vi "CreatePrivateEvents.vi"(8 "error in (no error)":errorcluster, 11 "SignalSenderLoop":refnum<class "SignalSenderLoop.lvclass">) -> (0 "error out":errorcluster, 3 "SignalSenderLoop out":refnum<class "SignalSenderLoop.lvclass">)   [LabVIEW 2020, in "SignalSenderLoop.lvclass"]
doc: "JKI State Machine Objects (SMO) 1.1.0.20\nJKI - JKI\nCopyright (c) 2016, JKI"
uses:
  SignalSenderLoop.lvclass
  SignalSenderLoop.lvclass/SignalSenderLoop.ctl
  Typedefs/AsyncMethodInputs--Cluster.ctl
  Typedefs/PrivateEvents--SignalSenderLoop.SignalCMDArry.ctl
  <vilib>/JKI/JKI SMO/SMO/SMO.lvclass
panel:
  # "For instructions on how to use the JKI State Machine Objects, examples and video tutorials, visit:\nhttp://jki.net/state-machine-objects/\n\nJKI State Machine Objects™\nhttp://jki.net/state-machine-objects/\nCopyright (C) 2005-2015, JKI <info@jki.net>\nALL RIGHTS RESERVED"
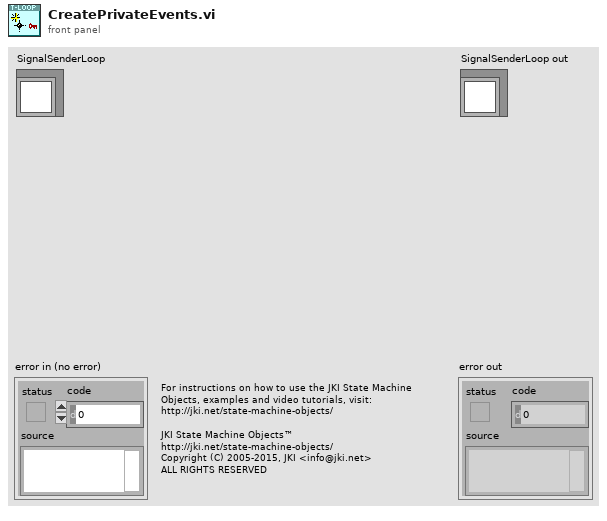
[diagram p1: front panel]
types:
  T1 = typedef "SignalSenderLoop.lvclass/PrivateData--Ref.ctl" = refnum<data-value>
  T2 = typedef "SignalSenderLoop.lvclass/PrivateEvents--SignalSenderLoop.SignalCMDArry.ctl" = dbl[]
  T3 = typedef "SignalSenderLoop.lvclass/AsyncMethodInputs--Cluster.ctl" = cluster{"Data":dbl}
  T4 = typedef "SignalSenderLoop.lvclass/PrivateData--Cluster.ctl" = cluster{"Public Events":T5, "Setpoint":T6, "Private Events":T7, "SignalFrameSet":T8}
  T5 = typedef "SignalSenderLoop.lvclass/PublicEvents--Cluster.ctl" = cluster{"Setpoint Changed":refnum<user-event>, "Value Changed":refnum<user-event>}
  T6 = typedef "SignalSenderLoop.lvclass/Data.ctl" = dbl
  T7 = typedef "SignalSenderLoop.lvclass/PrivateEvents--Cluster.ctl" = cluster{"AsyncMethod":refnum<user-event>, "SignalCMDArry":refnum<user-event>}
  T8 = typedef "SignalSenderLoop.lvclass/SignalFrameSet.ctl" = cluster{"Port_No.":refnum<k21>, "计数Count":bool, "校验CheckSum":bool, "MessageFrame":refnum<k21>, "校验算法名称":string}
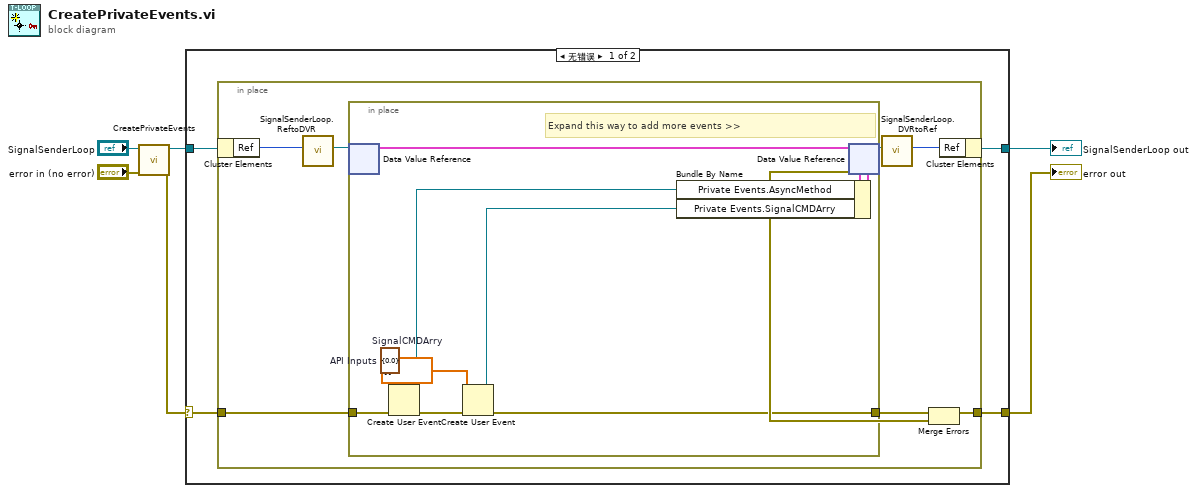
[diagram p0: block diagram]
diagram:
  n1 = call-parent "CreatePrivateEvents.vi"("error in (no error)"="error in (no error)", "SMO"="SignalSenderLoop") -> ("error out"=w4:errorcluster, "SMO out"=w2:refnum<class "SignalSenderLoop.lvclass">)  [unwired: 8 in]
  n2 = case shown="无错误" w4 {
    selector: w4 -> [w8 w29]
    tunnel: [w7 w29] -> w3
    tunnel: [w9 w28] -> w1
    tunnel: w2 -> [w10 w28]
    frame No Error {
      n3 = in-place {
        in-place-border: w8 -> [w18]
        in-place-border: [w15] -> w7
        n4 = in-place-cluster #1(w10) -> ("Ref"=w14:u32)
        n5 = call "SignalSenderLoop.ReftoDVR.vi"("Ref"=w14) -> ("Ref"=w13:T1)  [unwired: 10 in]
        n6 = in-place {
          in-place-border: w18 -> [w26]
          in-place-border: [w21] -> w17
          w20 = T2 []  # SignalCMDArry
          w23 = T3 {"Data"=0.0}  # API Inputs
          # "Expand this way to add more events >>"
          n7 = in-place-dvr #2(w13) -> (w25:T4)  [unwired: 1 out]
          n8 = Create User Event(user event datatype=w23, error in=w26) -> (user event=w24:refnum<user-event>, error out=w22:errorcluster)
          n9 = Create User Event(user event datatype=w20, error in=w22) -> (user event=w19:refnum<user-event>, error out=w21:errorcluster)
          n10 = Bundle By Name(cluster=w25, "Private Events.AsyncMethod"=w24, "Private Events.SignalCMDArry"=w19) -> (w27:T4)
          n11 = in-place-dvr #2(w27) -> (w12:T1, w16:errorcluster)
        }
        n12 = call "SignalSenderLoop.DVRtoRef.vi"("Ref"=w12) -> ("Ref"=w11:u32)  [unwired: 10 in]
        n13 = Merge Errors(w17, w16) -> (w15:errorcluster)
        n14 = in-place-cluster #1("Ref"=w11) -> (w9:refnum<class "SignalSenderLoop.lvclass">)
      }
    }
    frame Error {
    }
  }
  "error out" <- w3
  "SignalSenderLoop out" <- w1
